vi "Init_Keithley_4200.vi"(8 "error in (no error)":errorcluster, 11 "VISA resource name":refnum<visa-resource-name>) -> (0 "error out":errorcluster, 3 "VISA resource name out":refnum<visa-resource-name>)   [LabVIEW 2026]
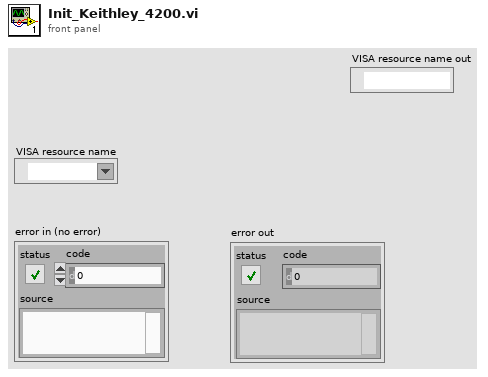
[diagram p1: front panel]
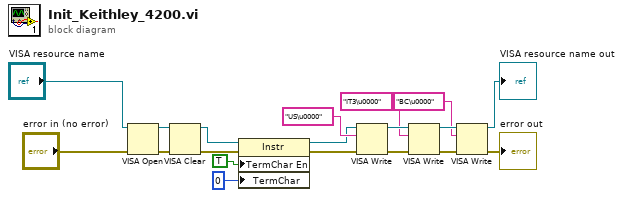
[diagram p0: block diagram]
diagram:
  n1 = VISA Open(error in (no error)="error in (no error)", VISA resource name="VISA resource name") -> (VISA resource name=w2:refnum<visa-resource-name>, error out=w3:errorcluster)  [unwired: 3 in]
  n2 = VISA Clear(VISA resource name=w2, error in (no error)=w3) -> (VISA resource name out=w7:refnum<visa-resource-name>, error out=w6:errorcluster)
  n3 = property class="Instr"(reference=w7, error in=w6, "TermChar En"=TRUE ("Message Based Settings:Termination Character Enable"), "TermChar"=u8 0 ("Message Based Settings:Termination Character")) -> (reference out=w9:refnum<visa-resource-name>, error out=w8:errorcluster)
  n4 = VISA Write(VISA resource name=w9, write buffer="US\u0000", error in (no error)=w8) -> (VISA resource name out=w17:refnum<visa-resource-name>, error out=w16:errorcluster)  [unwired: 1 out]
  n5 = VISA Write(VISA resource name=w17, write buffer="IT3\u0000", error in (no error)=w16) -> (VISA resource name out=w15:refnum<visa-resource-name>, error out=w14:errorcluster)  [unwired: 1 out]
  n6 = VISA Write(VISA resource name=w15, write buffer="BC\u0000", error in (no error)=w14) -> (VISA resource name out=→"VISA resource name out":refnum<visa-resource-name>, error out=→"error out":errorcluster)  [unwired: 1 out]
